vi "Parameters_BuildPositionMove.vi"(8 "Acceleration Jerk":dbl=1000.0, 9 "Acceleration":dbl=10000.0, 10 "Velocity":dbl=1000.0, 11 "Target Position":dbl) -> (3 "Parameters":dbl[](array[numeric]))   [LabVIEW 2017, in "WordManipulationLibrary.lvlib"]
uses:
  WordManipulationLibrary.lvlib
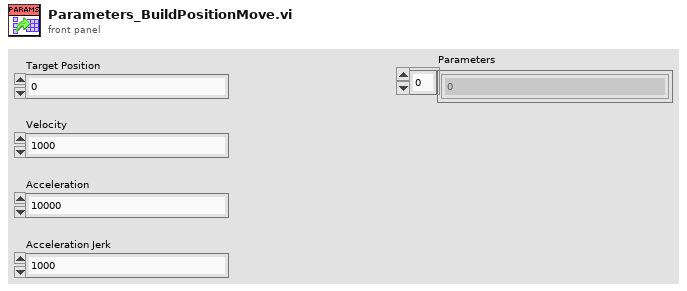
[diagram p1: front panel]
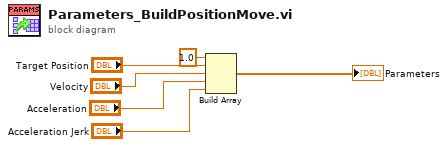
[diagram p0: block diagram]
diagram:
  n1 = Build Array(1.0 ("element"), "Target Position", "Velocity", "Acceleration", "Acceleration Jerk") -> (→"Parameters":dbl[])
